vi "GetText.vi"(8 "error in":errorcluster, 11 "channel in":refnum<class "channel node.lvclass">) -> (0 "error out":errorcluster, 1 "additional text":string, 2 "text":string, 3 "channel out":refnum<class "channel node.lvclass">, 4 "glyph":string)   [LabVIEW 2013, in "channel node.lvclass"]
uses:
  channel node.lvclass
  channel node.lvclass/channel node.ctl
  channel configuration/channel configuration.lvclass/channel configuration.ctl
  channel configuration/channel configuration.lvclass
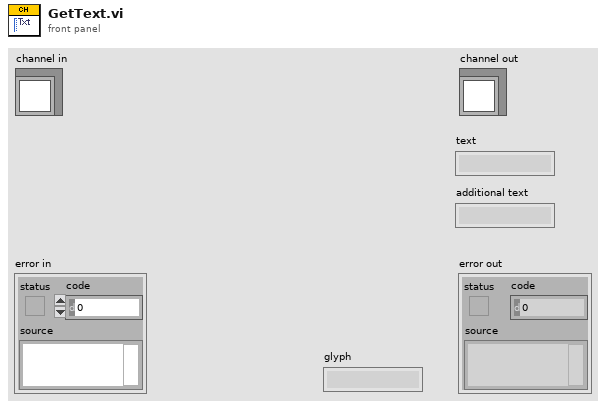
[diagram p1: front panel]
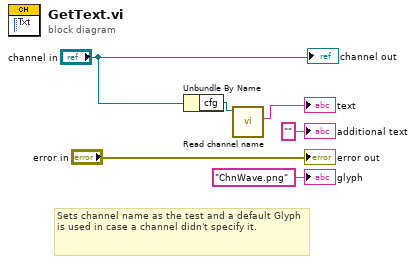
[diagram p0: block diagram]
diagram:
  # "Sets channel name as the test and a default Glyph is used in case a channel didn't specify it."
  n1 = Unbundle By Name("channel in") -> ("cfg"=w2:refnum<class "channel configuration.lvclass">)
  n2 = call "Read channel name.vi"("channel config object in"=w2) -> ("channel name"=→"text":string)  [unwired: 8 in, 2 out]
  "error out" <- "error in"
  "channel out" <- "channel in"
  "additional text" <- "" ("additional text")
  "glyph" <- "ChnWave.png" ("glyph")
